vi "_s_IEEE754formatReverse.vi"(8 "error in (no error)":errorcluster, 9 "Number":sgl=-101.101 format="%.2f") -> (0 "error out":errorcluster, 1 "String":string="459CFFAE")   [LabVIEW 2013]
doc: "This VI shows how LabVIEW stores SGL floating-point numbers in memory in binary format. The 32-bit binary number is based on the following IEEE 754 format:\n\n1 bit for the SIGN\n8 bits for the EXPONENT\n23 bits for the MANTISSA\n\nThe formula for the conversion is the following:\n\nSGL = (-1)^SIGN * 1.MANTISSA * 2^(EXPONENT-127)\n\nYou can use this VI to convert SGL numbers to their binary storage equivalent, and vice versa."
panel:
  # "SGL to Binary Storage Format"
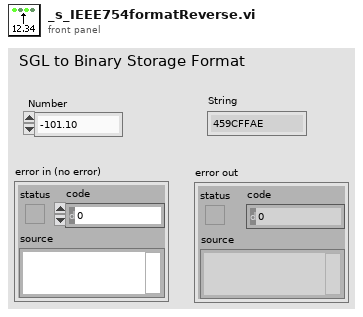
[diagram p1: front panel]
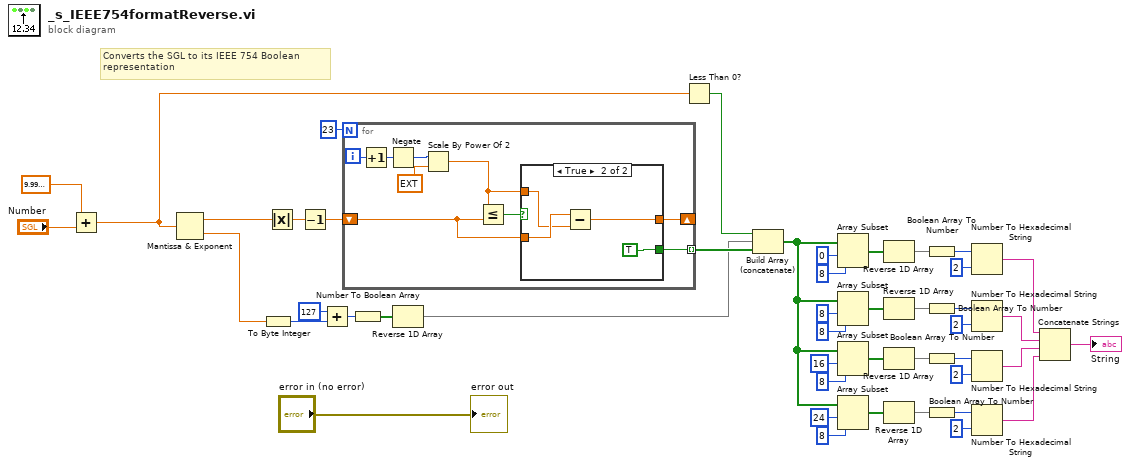
[diagram p0: block diagram]
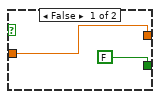
[diagram p2: hidden frame]
diagram:
  # "Converts the SGL to its IEEE 754 Boolean \nrepresentation"
  n1 = Add(x=sgl 1e-06, y="Number") -> (x+y=w2:sgl)
  n2 = Mantissa & Exponent(0:w2) -> (1:w37:sgl, 2:w40:sgl)
  n3 = To Byte Integer(number=w40) -> (8bit integer=w46:i8)
  n4 = Absolute Value(x=w37) -> (abs(x)=w38:sgl)
  n5 = Decrement(x=w38) -> (x-1=w42:sgl)
  n6 = Add(x=i8 127, y=w46) -> (x+y=w45:i8)
  n7 = for {
    N: 23 -> [_]
    shift-right: [w48] -> _
    shift-left: w42 -> [w50]
    tunnel: [w47] -> w35 mode=indexing
    i -> [w55]
    n8 = Increment(x=w55) -> (x+1=w54:i32)
    n9 = Negate(x=w54) -> (-x=w53:i32)
    n10 = Scale By Power Of 2(n=w53, x=ext 1.0) -> (x*2^n=w49:ext)
    n11 = Less Or Equal?(x=w49, y=w50) -> (x <= y?=w51:bool)
    n12 = case shown="True" w51 {
      tunnel: w50 -> [w56 w61]
      tunnel: w49 -> [_ w58]
      tunnel: [w56 w60] -> w48
      tunnel: [FALSE TRUE] -> w47
      frame False {
      }
      frame True {
        n13 = Subtract(x=w61, y=w58) -> (x-y=w60:ext)
      }
    }
  }
  n14 = Number To Boolean Array(number=w45) -> (Boolean array=w44:bool[])
  n15 = Reverse 1D Array(array=w44) -> (reversed array=w34:bool[])
  n16 = Less Than 0?(x=w2) -> (x < 0?=w36:bool)
  n17 = Build Array (concatenate)(w36, w34, w35) -> (w7:bool[])
  n18 = Array Subset(array=w7, index=0, length=8) -> (w24:bool[])
  n19 = Array Subset(array=w7, index=8, length=8) -> (w19:bool[])
  n20 = Array Subset(array=w7, index=16, length=8) -> (w17:bool[])
  n21 = Array Subset(array=w7, index=24, length=8) -> (w15:bool[])
  n22 = Reverse 1D Array(array=w24) -> (reversed array=w6:bool[])
  n23 = Reverse 1D Array(array=w19) -> (reversed array=w5:bool[])
  n24 = Reverse 1D Array(array=w17) -> (reversed array=w4:bool[])
  n25 = Reverse 1D Array(array=w15) -> (reversed array=w3:bool[])
  n26 = Boolean Array To Number(Boolean array=w6) -> (number=w23:u32)
  n27 = Boolean Array To Number(Boolean array=w5) -> (number=w20:u32)
  n28 = Boolean Array To Number(Boolean array=w4) -> (number=w18:u32)
  n29 = Boolean Array To Number(Boolean array=w3) -> (number=w16:u32)
  n30 = Number To Hexadecimal String(1:i16 2 ("width (-)"), 2:w23) -> (0:w22:string)
  n31 = Number To Hexadecimal String(1:i16 2 ("width (-)"), 2:w20) -> (0:w14:string)
  n32 = Number To Hexadecimal String(1:i16 2 ("width (-)"), 2:w18) -> (0:w13:string)
  n33 = Number To Hexadecimal String(1:i16 2 ("width (-)"), 2:w16) -> (0:w12:string)
  n34 = Concatenate Strings(w22, w14, w13, w12) -> (→"String":string)
  "error out" <- "error in (no error)"
